vi "cluster_v33.vi"() -> ()   [LabVIEW 2009]
uses:
  <vilib>/Math Plots/3D Math Plots/3D Surface/3D Surface XCtrl/3D Surface.xctl
  <vilib>/Math Plots/3D Math Plots/3D Surface/3D Surface Datatype/3D Surface Datatype.lvclass
  <vilib>/Math Plots/3D Math Plots/3D Surface/3D Surface Datatype/Public/Plot Helper (Vector).vi
  <vilib>/Analysis/Matrix/Numeric/Conversions/Array To Matrix - RA2.vi
  <vilib>/Analysis/Matrix/NI_Matrix.lvlib
panel:
  in  "eps":dbl(slide)=68.57142857142857 scale=0.0..80.0
  in  "sig":dbl(slide)=0.9721115537848606 scale=0.0..2.0
  out "3D Surface":refnum<class "3D Plot Datatype.lvclass">[](xcontrol)
  out "X":dbl=19.324110671936744
  out "y":dbl=19.324110671936744
  in  "stop":bool
  in  "Domeniul de definitie x,y":dbl(slide)=38.648221343873516 scale=0.5..100.0
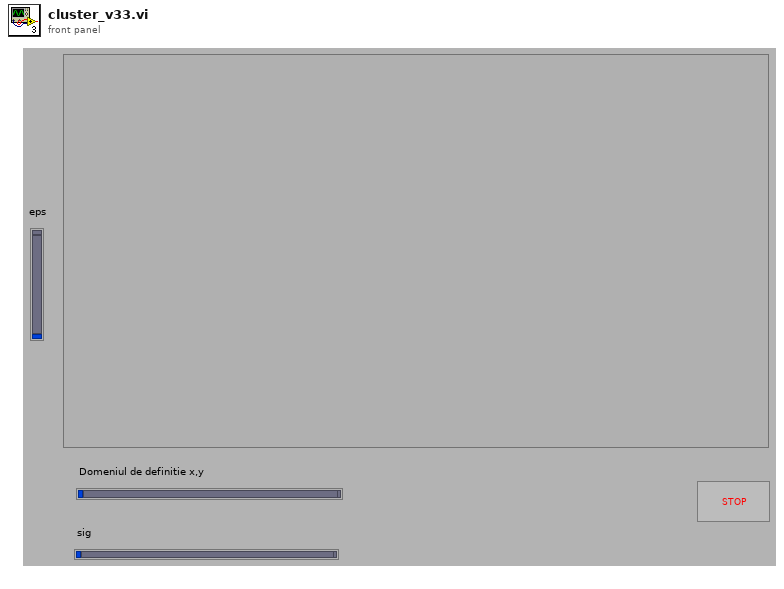
[diagram p1: front panel]
types:
  T1 = typedef "NI_Matrix.lvlib/RealMatrix.ctl" = dbl[][]
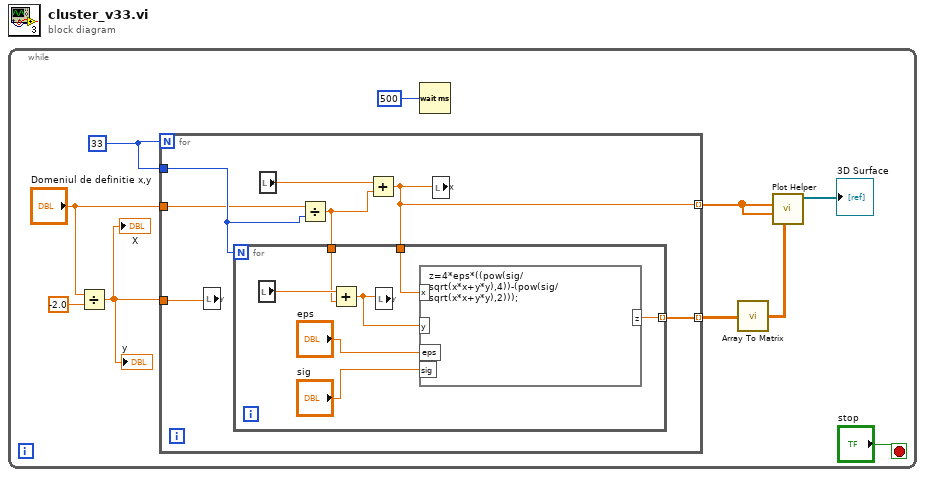
[diagram p0: block diagram]
diagram:
  n1 = while {
    stop <- "stop" stop-if-true
    w4 = 33
    n2 = Divide(x="Domeniul de definitie x,y", y=-2.0) -> (x/y=w1:dbl)
    "X" <- w1
    "y" <- w1
    n3 = for {
      N: w4 -> [_]
      tunnel: [w16] -> w8 mode=indexing
      tunnel: [w15] -> w9 mode=indexing
      tunnel: w4 -> [w14]
      tunnel: w1 -> [w12]
      tunnel: "Domeniul de definitie x,y" -> [w11]
      n4 = local write "y"(w12) -> ()
      n5 = local read "X"() -> (w17:dbl)
      n6 = Divide(x=w11, y=w14) -> (x/y=w13:dbl)
      n7 = Add(x=w17, y=w13) -> (x+y=w16:dbl)
      n8 = for {
        N: w14 -> [_]
        tunnel: w16 -> [w23]
        tunnel: [w21] -> w15 mode=indexing
        tunnel: w13 -> [w20]
        n9 = local read "y"() -> (w24:dbl)
        n10 = Add(x=w24, y=w20) -> (x+y=w22:dbl)
        n11 = local write "y"(w22) -> ()
        n12 = formula code="z=4*eps*((pow(sig/sqrt(x*x+y*y),4))-(pow(sig/sqrt(x*x+y*y),2)));"("x"=w23, "y"=w22, "eps"="eps", "sig"="sig") -> ("z"=w21:dbl)
      }
      n13 = local write "X"(w16) -> ()
    }
    n14 = Wait (ms)(milliseconds to wait=500) -> ()  [unwired: 1 out]
    n15 = call-poly <vilib>:"Array To Matrix.vi"("Real 2D Array"=w9) -> ("Real Matrix"=w10:T1)
    n16 = call-poly <vilib>:"Plot Helper.vi"("z matrix"=w10, "y vector"=w8, "x vector"=w8) -> ("3D Plot lvclass Array out"=→"3D Surface":refnum<class "3D Plot Datatype.lvclass">[])  [unwired: 3 in, 5 out]
  }
